vi "Thorlabs MC2000B Read & Write demo.vi"() -> ()   [LabVIEW 2013]
doc: "This example shows how to acquire a power measurement using the VIs of the driver."
uses:
  <instrlib>/Thorlabs_MC2000B/Public/Advanced/Blade.ctl
  <instrlib>/Thorlabs_MC2000B/Public/Advanced/Output mode.ctl
  <instrlib>/Thorlabs_MC2000B/Public/Advanced/Reference Mode_High Precision.ctl
  <instrlib>/Thorlabs_MC2000B/Public/Advanced/Reference Mode.ctl
  <instrlib>/Thorlabs_MC2000B/Thorlabs_MC2000B.lvlib
panel:
  out "Mode":T1(tab)
  in  "High Precision Reference Mode":T2
  out "High Precision Reference Mode Read":T3(ring)
  in  "Reference Mode":T4
  out "Reference Mode Read":T4
  out "Reference out Frequency (Hz)":i32
  out "Output":T5
  in  "Actual?":T5
  out "Blade Type Read":T6=enum."MC1F10"
  in  "Blade Type":T6
  out "Enabled?":bool
  in  "Enable":bool=TRUE
  out "Frequence Read":i32=20
  in  "Frequence (Hz)":i32=20
  out "COM Ports":string[](array[string])=["COM1", "COM17", "COM19"]
  # "(c) 2016 <Thorlabs>.  ALL RIGHTS RESERVED."
  # "Connect"
  # "Set data"
  # "Read data"
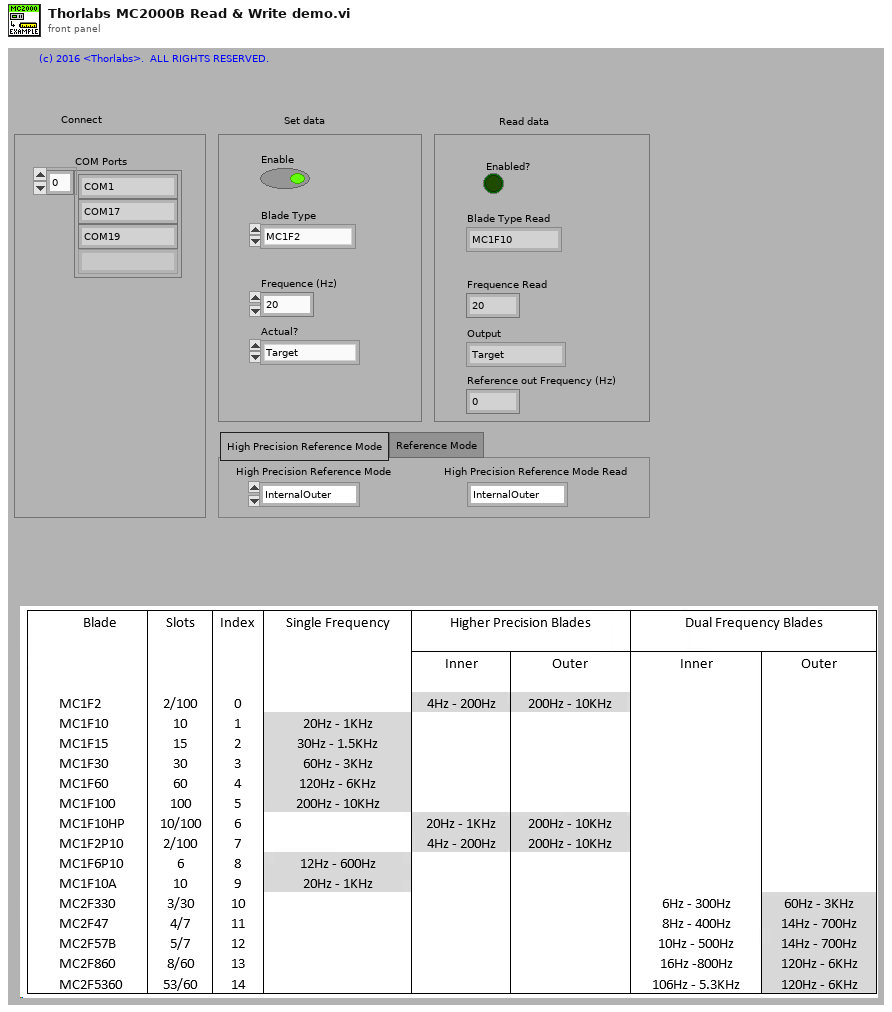
[diagram p1: front panel]
types:
  T1 = enum32{"High Precision Reference Mode", "Reference Mode"}
  T2 = typedef "Thorlabs_MC2000B.lvlib/Reference Mode_High Precision.ctl" = enum16{"InternalOuter", "InternalInner", "ExternalOuter", "ExternalInner"}
  T3 = enum16{"InternalOuter", "InternalInner", "ExternalOuter", "ExternalInner"}
  T4 = typedef "Thorlabs_MC2000B.lvlib/Reference Mode.ctl" = enum16{"Internal", "External"}
  T5 = typedef "Thorlabs_MC2000B.lvlib/Output mode.ctl" = enum16{"Target", "Actual/Outer", "Inner", "Sum", "Diff"}
  T6 = typedef "Thorlabs_MC2000B.lvlib/Blade.ctl" = enum16{"MC1F2", "MC1F10", "MC1F15", "MC1F30", "MC1F60", "MC1F100", "MC1F10HP", "MC1F2P10", "MC1F6P10", "MC1F10A", "MC2F330", "MC2F47", "MC2F57B", "MC2F860", "MC2F5360"}
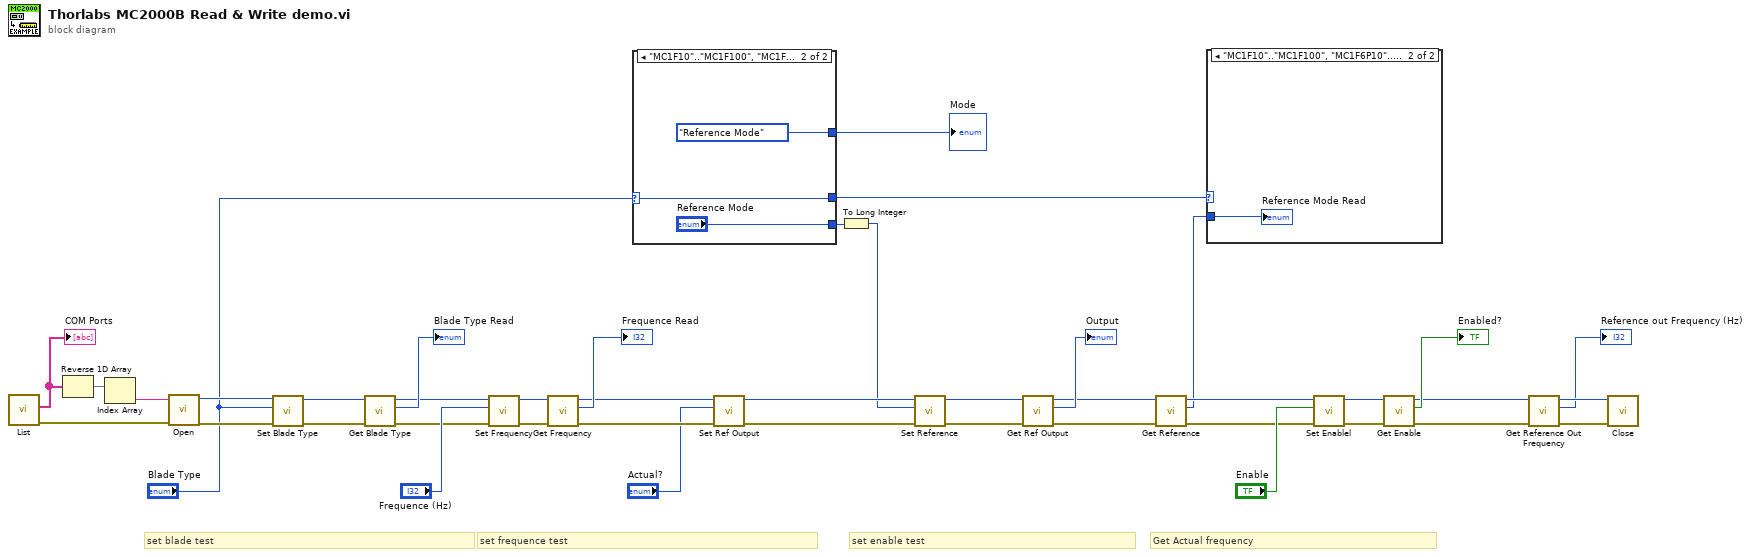
[diagram p0: block diagram]
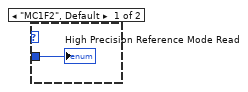
[diagram p2: hidden frame]
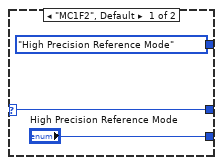
[diagram p3: hidden frame]
diagram:
  # "Get Actual frequency"
  # "set frequence test"
  # "set blade test"
  # "set enable test"
  n1 = call <instrlib>:"List.vi"() -> ("error out"=w39:errorcluster, "Serial Ports"=w42:string[])  [unwired: 8 in, 2 out]
  "COM Ports" <- w42
  n2 = Reverse 1D Array(array=w42) -> (reversed array=w41:string[])
  n3 = Index Array(array=w41) -> (element=w40:string)  [unwired: 1 in]
  n4 = call <instrlib>:"Open.vi"("error in (no error)"=w39, "Serial Port"=w40) -> ("error out"=w17:errorcluster, "Handle out"=w18:i32)  [unwired: 7 in, 1 out]
  n5 = call <instrlib>:"Set Blade Type.vi"("error in (no error)"=w17, "Blade Type"="Blade Type", "Handle in"=w18) -> ("error out"=w23:errorcluster, "Handle out"=w24:i32)  [unwired: 7 in]
  n6 = call <instrlib>:"Get Blade Type.vi"("error in (no error)"=w23, "Handle in"=w24) -> ("error out"=w25:errorcluster, "Blade Type"=→"Blade Type Read":T6, "Handle out"=w26:i32)  [unwired: 7 in]
  n7 = call <instrlib>:"Set Frequency.vi"("error in (no error)"=w25, "Frequency (Hz)"="Frequence (Hz)", "Handle in"=w26) -> ("error out"=w29:errorcluster, "Handle out"=w28:i32)  [unwired: 7 in]
  n8 = call <instrlib>:"Get Frequency.vi"("error in (no error)"=w29, "Handle in"=w28) -> ("error out"=w33:errorcluster, "Frequency (Hz)"=→"Frequence Read":i32, "Handle out"=w34:i32)  [unwired: 7 in]
  n9 = case shown="\"MC1F10\"..\"MC1F100\", \"MC1F6P10\"..\"MC2F5360\"" "Blade Type" {
    selector: "Blade Type" -> [w43 w46]
    tunnel: ["High Precision Reference Mode" "Reference Mode"] -> w10
    tunnel: [T1."High Precision Reference Mode" ("Mode") T1."Reference Mode" ("Mode")] -> w5
    tunnel: [w43 w46] -> w3
    frame "MC1F2", Default {
    }
    frame "MC1F10".."MC1F100", "MC1F6P10".."MC2F5360" {
    }
  }
  "Mode" <- w5
  n10 = call <instrlib>:"Set Ref Output.vi"("error in (no error)"=w33, "Actual?"="Actual?", "Handle in"=w34) -> ("error out"=w12:errorcluster, "Handle out"=w14:i32)  [unwired: 7 in]
  n11 = To Long Integer(number=w10) -> (32bit integer=w1:i32)
  n12 = call <instrlib>:"Set Reference.vi"("error in (no error)"=w12, "Reference Mode"=w1, "Handle in"=w14) -> ("error out"=w11:errorcluster, "Handle out"=w13:i32)  [unwired: 7 in]
  n13 = call <instrlib>:"Get Ref Output.vi"("error in (no error)"=w11, "Handle in"=w13) -> ("error out"=w7:errorcluster, "Output"=→"Output":T5, "Handle out"=w9:i32)  [unwired: 7 in]
  n14 = call <instrlib>:"Get Reference.vi"("error in (no error)"=w7, "Handle in"=w9) -> ("error out"=w6:errorcluster, "Reference Type"=w2:i32, "Handle out"=w8:i32)  [unwired: 7 in]
  n15 = case shown="\"MC1F10\"..\"MC1F100\", \"MC1F6P10\"..\"MC2F5360\"" w3 {
    tunnel: w2 -> [w49 w50]
    frame "MC1F2", Default {
      "High Precision Reference Mode Read" <- w49
    }
    frame "MC1F10".."MC1F100", "MC1F6P10".."MC2F5360" {
      "Reference Mode Read" <- w50
    }
  }
  n16 = call <instrlib>:"Set Enablel.vi"("error in (no error)"=w6, "Enable?"="Enable", "Handle in"=w8) -> ("error out"=w21:errorcluster, "Handle out"=w22:i32)  [unwired: 7 in]
  n17 = call <instrlib>:"Get Enable.vi"("error in (no error)"=w21, "Handle in"=w22) -> ("error out"=w15:errorcluster, "Enable?"=→"Enabled?":bool, "Handle out"=w16:i32)  [unwired: 7 in]
  n18 = call <instrlib>:"Get Reference Out Frequency.vi"("error in (no error)"=w15, "Handle in"=w16) -> ("error out"=w38:errorcluster, "Reference out Frequency (Hz)"=→"Reference out Frequency (Hz)":i32, "Handle out"=w37:i32)  [unwired: 7 in]
  n19 = call <instrlib>:"Close.vi"("error in (no error)"=w38, "hdl"=w37) -> ()  [unwired: 9 in, 1 out]
